vi "Read_Write_Trav_position.vi"(2 "Channel Properties":T1[](array[typedef]) {"Current Pos" format="%.2f"; "Backlash/Eng units" format="%.2f"; "Pulses/rev" format="%.2f"; "Pos Tolerance" format="%.2f"; "Pulses/unit" format="%.2f"; "Acc. Min" format="%.2f"; "Acc. Max" format="%.2f"; "Vel. Min" format="%.2f"; "Vel. Max" format="%.2f"; "Acc. Default" format="%.2f"; "Vel. Default" format="%.2f"}, 3 "Mode":T2(ring), 4 "Traverse Name":string="EnFlo Tunnel") -> (0 "Channel Properties Out":T1[](array[typedef]) {"Current Pos" format="%.2f"; "Backlash/Eng units" format="%.2f"; "Pulses/rev" format="%.2f"; "Pos Tolerance" format="%.2f"; "Pulses/unit" format="%.2f"; "Acc. Min" format="%.2f"; "Acc. Max" format="%.2f"; "Vel. Min" format="%.2f"; "Vel. Max" format="%.2f"; "Acc. Default" format="%.2f"; "Vel. Default" format="%.2f"})   [LabVIEW 2022 SP3]
uses:
  Anemometry/Anemometry Sub Vis/Globals/Constants_global.vi
  DriveConfigGlobal.vi
  DriveProperties.ctl
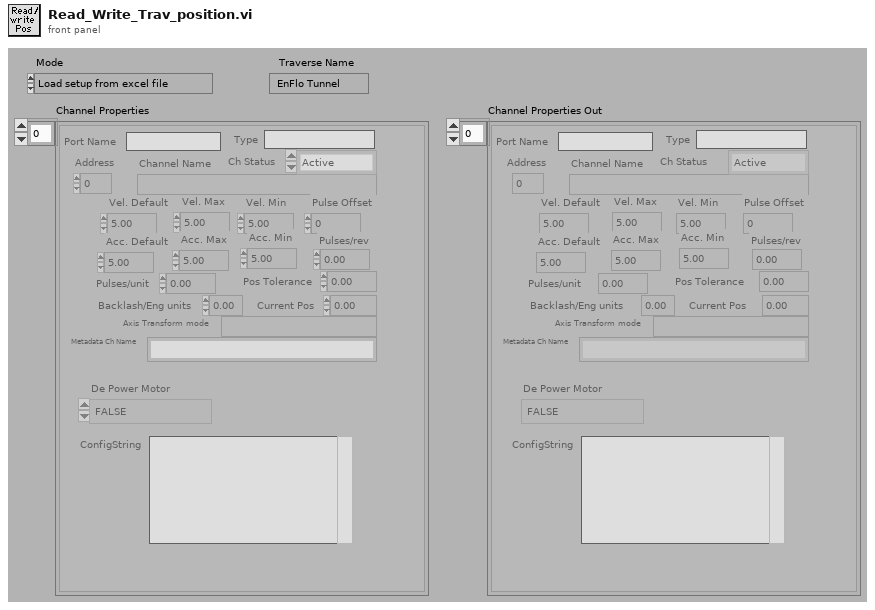
[diagram p1: front panel]
types:
  T1 = typedef "DriveProperties.ctl" = cluster{"Channel Name":string, "Vel. Default":sgl, "Acc. Default":sgl, "Vel. Max":sgl, "Vel. Min":sgl, "Acc. Max":sgl, "Acc. Min":sgl, "Pulses/unit":sgl, "Address":u8, "Pulse Offset":i32, "Pos Tolerance":sgl, "Pulses/rev":sgl, "Backlash/Eng units":sgl, "Current Pos":sgl, "Ch Status":enum16{"Active", "Offline", "Simulate"}, "Port Name":string, "Axis Transform mode":string, "Metadata Ch Name":string, "Type":string, "De Power Motor":enum16{"TRUE", "FALSE"}, "ConfigString":string}
  T2 = enum16{"Load setup from excel file", "Save setup to excel file"}
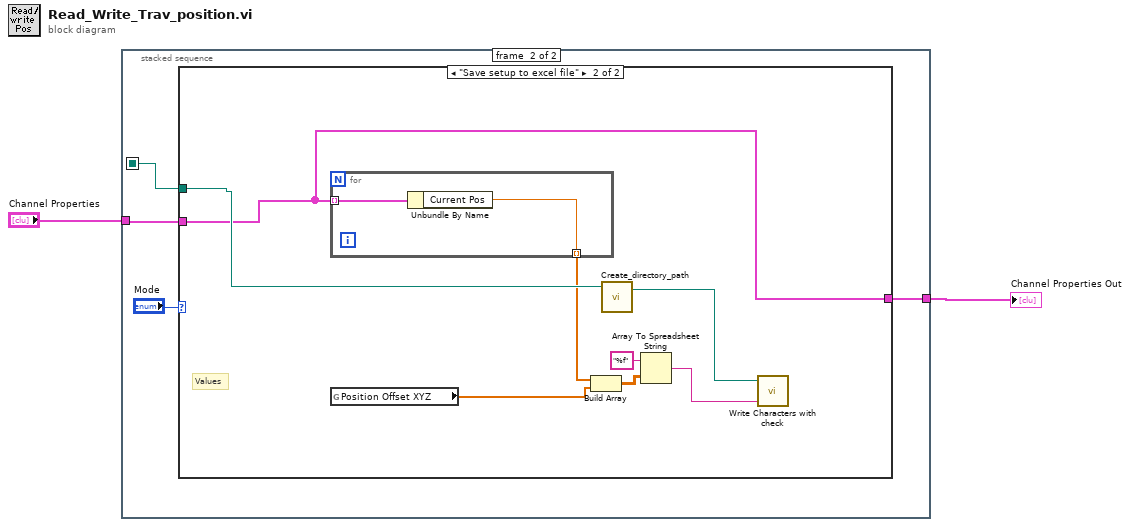
[diagram p0: block diagram]
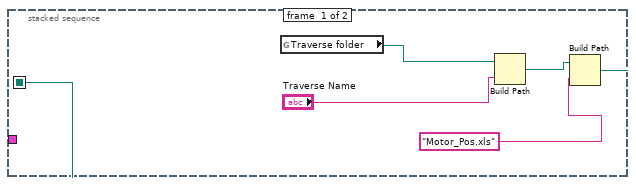
[diagram p2: hidden frame]
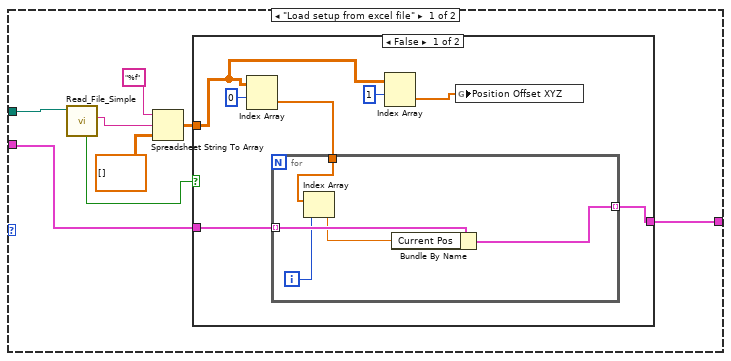
[diagram p3: hidden frame]
diagram:
  n1 = stacked-sequence {
    seq-local: [w4 _] -> [_ w10]
    tunnel: "Channel Properties" -> [_ w9]
    tunnel: [_ w8] -> w1
    frame #0 {
      n2 = global read "Constants_global.vi" "Traverse folder"() -> (w5:path)
      n3 = Build Path(base path=w5, name or relative path="Traverse Name") -> (appended path=w3:path)
      n4 = Build Path(base path=w3, name or relative path="Motor_Pos.xls" ("Substring")) -> (appended path=w4:path)
    }
    frame #1 {
      n5 = case shown="\"Save setup to excel file\"" "Mode" {
        tunnel: w10 -> [w19 w39]
        tunnel: w9 -> [w18 w38]
        tunnel: [w17 w38] -> w8
        frame "Load setup from excel file" {
          n6 = call "Read_File_Simple.vi"("Filename"=w19) -> ("Error?"=w13:bool, "string"=w14:string)  [unwired: 2 in, 6 out]
          n7 = Spreadsheet String To Array(format string="%f", spreadsheet string=w14, array type (2D Dbl)=dbl[][] []) -> (array=w12:dbl[][])  [unwired: 1 out]
          n8 = case shown="False" w13 {
            tunnel: w18 -> [w26 w32]
            tunnel: [w25 w32] -> w17
            tunnel: w12 -> [w21 _]
            frame False {
              n9 = Index Array(array=w21, index (row)=0) -> (element=w23:dbl[])  [unwired: 1 in]
              n10 = for {
                tunnel: w26 -> [w31] mode=indexing
                tunnel: [w30] -> w25 mode=indexing
                tunnel: w23 -> [w29]
                i -> [w28]
                n11 = Index Array(array=w29, index=w28) -> (element=w27:dbl)
                n12 = Bundle By Name(cluster=w31, "Current Pos"=w27) -> (w30:T1)
              }
              n13 = Index Array(array=w21, index (row)=1) -> (element=w20:dbl[])  [unwired: 1 in]
              n14 = global write "DriveConfigGlobal.vi" "Position Offset XYZ"(w20) -> ()
            }
            frame True {
            }
          }
        }
        frame "Save setup to excel file" {
          # "Values"
          n15 = for {
            tunnel: w38 -> [w42] mode=indexing
            tunnel: [w41] -> w37 mode=indexing
            n16 = Unbundle By Name(w42) -> ("Current Pos"=w41:sgl)
          }
          n17 = global read "DriveConfigGlobal.vi" "Position Offset XYZ"() -> (w36:dbl[])
          n18 = Build Array(w37, w36) -> (w35:dbl[][])
          n19 = call "Create_directory_path.vi"("Path name"=w39) -> ("Path name Out"=w34:path)  [unwired: 2 in, 1 out]
          n20 = Array To Spreadsheet String(array=w35, 3:"%f" ("format string")) -> (spreadsheet string=w33:string)  [unwired: 1 out]
          n21 = call "Write Characters with check.vi"("String to Write"=w33, "file (use dialog)"=w34) -> ()  [unwired: 2 in, 1 out]
        }
      }
    }
  }
  "Channel Properties Out" <- w1
